vi "Release VISA Lock.vi"(8 "error in (no error)":errorcluster, 11 "VISA resource name":refnum<visa-resource-name>) -> (0 "error out":errorcluster, 3 "VISA resource name out":refnum<visa-resource-name>)   [LabVIEW 2021, in "MB_VISA_Lock.lvlib"]
doc: "Releases this session's exclusive lock on the VISA resource.\n\nInput errors do not affect the behavior of this VI."
uses:
  <vilib>/Plasmionique/MB Master/MB_VISA_Lock/MB_VISA_Lock.lvlib
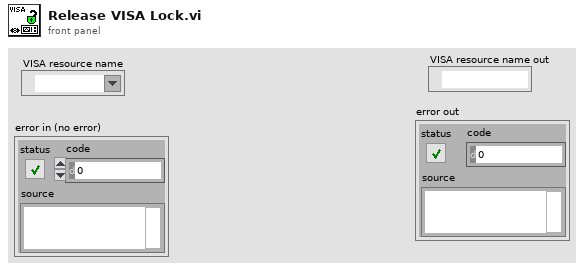
[diagram p1: front panel]
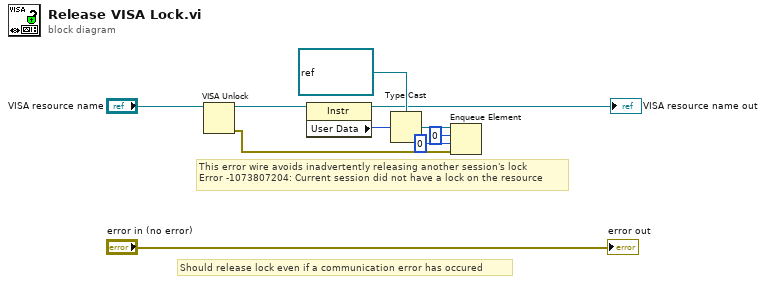
[diagram p0: block diagram]
diagram:
  # "This error wire avoids inadvertently releasing another session's lock\nError -1073807204: Current session did not have a lock on the resource"
  # "Should release lock even if a communication error has occured"
  n1 = VISA Unlock(11:"VISA resource name") -> (0:w1:errorcluster, 3:w4:refnum<visa-resource-name>)  [unwired: 1 in]
  n2 = property class="Instr"(reference=w4) -> (reference out=→"VISA resource name out":refnum<visa-resource-name>, "User Data"=w8:u32)  [unwired: 1 in, 1 out]
  n3 = Type Cast(type=refnum<queue> refnum ("lock ref in"), x=w8) -> (*(type *) &x=w6:refnum<queue>)
  n4 = Enqueue Element(queue=w6, element=0, timeout in ms (-1)=0, error in (no error)=w1) -> ()  [unwired: 3 out]
  "error out" <- "error in (no error)"
